vi "FormMain.vi"() -> ()   [LabVIEW 2018]
panel:
  out "String (transparent)":string
  in  "Vertical Add Button":bool
  in  "Vertical Open Button":bool
  in  "Vertical Stop Button":bool
  in  "Vertical Start Button":bool
  out "滑动杆":u8(slide) max=1 scale=0.0..15.0
  in  "TDMS Files Path":path
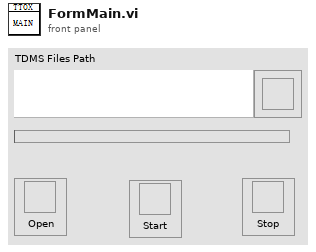
[diagram p1: front panel]
types:
  T1 = enum8{"Enabled", "Disabled", "Disabled and Grayed Out"}
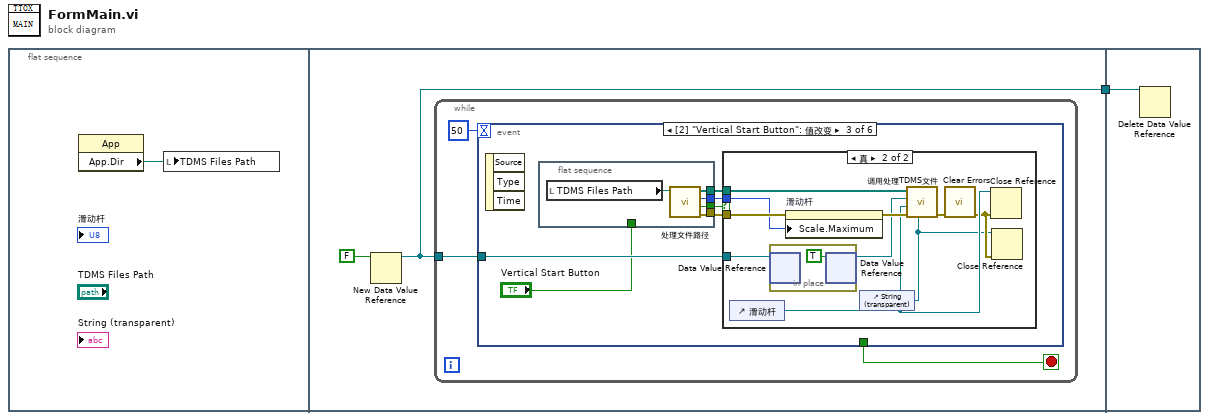
[diagram p0: block diagram]
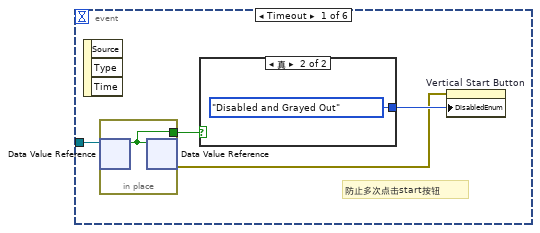
[diagram p2: hidden frame]
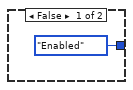
[diagram p3: hidden frame]
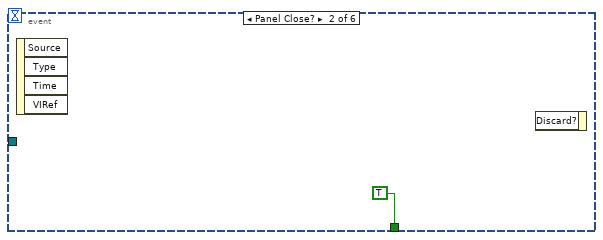
[diagram p4: hidden frame]
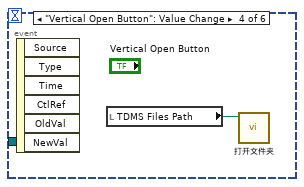
[diagram p6: hidden frame]
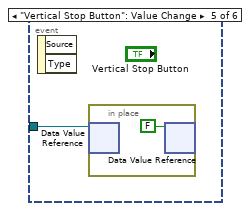
[diagram p7: hidden frame]
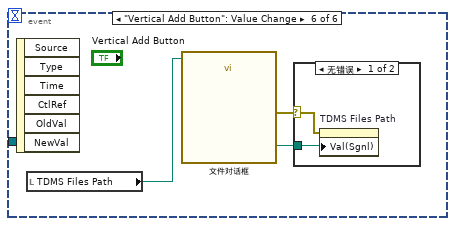
[diagram p8: hidden frame]
diagram:
  n1 = flat-sequence {
    tunnel: [w3] -> w1
    tunnel: w1 -> [w46]
    frame #0 {
      n2 = property class="App"() -> ("App.Dir"=w2:path)  [unwired: 2 in, 2 out]
      n3 = local write "TDMS Files Path"(w2) -> ()
    }
    frame #1 {
      n4 = New Data Value Reference(data value=FALSE) -> (data value reference=w3:refnum<data-value>)  [unwired: 1 in, 1 out]
      n5 = while {
        tunnel: w3 -> [w7]
        stop <- w6 stop-if-true
        n6 = event shown="[2] \"Vertical Start Button\": 值改变" {
          selector: _ -> [_ _ _ _ _ _]
          dyn-events: _ -> [_ _ _ _ _ _]
          timeout: 50 -> [_ _ _ _ _ _]
          tunnel: w7 -> [w11 _ w18 _ w39 _]
          tunnel: [_ TRUE _ _ _ _] -> w6
          event Timeout {
            # "防止多次点击start按钮"
            n7 = event-data() -> ()  [unwired: 1 in, 3 out]
            n8 = in-place {
              in-place-border: [w14] -> w10
              n9 = in-place-dvr #1(w11) -> (w14:bool)  [unwired: 1 out]
              n10 = in-place-dvr #1(w14) -> (w8:errorcluster)  [unwired: 1 out]
            }
            n11 = case shown="真" w10 {
              tunnel: [T1."Enabled" ("禁用") T1."Disabled and Grayed Out" ("禁用")] -> w9
              frame False {
              }
              frame True {
              }
            }
            n12 = property on="Vertical Start Button" class="Bool"(error in=w8, "DisabledEnum"=w9) -> ()  [unwired: 1 in, 2 out]
          }
          event Panel Close? {
            n13 = event-data() -> ()  [unwired: 1 in, 4 out]
            n14 = event-data() -> ()  [unwired: 2 in, 1 out]
          }
          event "Vertical Start Button": Value Change {
            n15 = event-data() -> ()  [unwired: 1 in, 3 out]
            n16 = flat-sequence {
              tunnel: [w25] -> w21
              tunnel: [w24] -> w20
              tunnel: [w23] -> w19
              tunnel: "Vertical Start Button" -> [_]
              tunnel: [w22] -> w16
              frame #0 {
                n17 = local read "TDMS Files Path"() -> (w26:path)
                n18 = call "处理文件路径.vi"("TDMS Files Path"=w26) -> ("错误输出"=w24:errorcluster, "可用"=w25:bool, "文件个数"=w22:i32, "文件数组"=w23:path[])  [unwired: 7 in]
              }
            }
            n19 = case shown="真" w21 {
              tunnel: w20 -> [_ w36]
              tunnel: w19 -> [_ w35]
              tunnel: w18 -> [_ w33]
              tunnel: w16 -> [_ w30]
              frame False {
              }
              frame True {
                n20 = control-ref of="滑动杆"() -> (w29:refnum<vi>)
                n21 = in-place {
                  n22 = in-place-dvr #2(w33) -> ()  [unwired: 2 out]
                  n23 = in-place-dvr #2(TRUE ("数据值")) -> (w32:refnum<data-value>)  [unwired: 1 out]
                }
                n24 = property on="滑动杆" class="Slide (严格)"(error in=w36, "Scale.Maximum"=w30) -> (error out=w34:errorcluster)  [unwired: 1 in, 1 out]
                n25 = control-ref of="String (transparent)"() -> (w27:refnum<vi>)
                n26 = call "调用处理TDMS文件.vi"("String"=w27, "error in (no error)"=w34, "滑动杆引用"=w29, "停止引用"=w32, "文件路径数组"=w35) -> ("error out"=w31:errorcluster)  [unwired: 6 in]
                n27 = call <vilib>:"Clear Errors.vi"("error in (no error)"=w31) -> ("error out"=w28:errorcluster)  [unwired: 5 in, 1 out]
                n28 = Close Reference(reference=w29, error in (no error)=w28) -> ()  [unwired: 1 out]
                n29 = Close Reference(reference=w27, error in (no error)=w28) -> ()  [unwired: 1 out]
              }
            }
          }
          event "Vertical Open Button": Value Change {
            n30 = event-data() -> ()  [unwired: 1 in, 6 out]
            n31 = local read "TDMS Files Path"() -> (w38:path)
            n32 = call "打开文件夹.vi"("文件夹"=w38) -> ()  [unwired: 10 in, 1 out]
          }
          event "Vertical Stop Button": Value Change {
            n33 = event-data() -> ()  [unwired: 1 in, 2 out]
            n34 = in-place {
              n35 = in-place-dvr #3(w39) -> ()  [unwired: 2 out]
              n36 = in-place-dvr #3(FALSE ("数据值")) -> ()  [unwired: 2 out]
            }
          }
          event "Vertical Add Button": Value Change {
            n37 = event-data() -> ()  [unwired: 1 in, 6 out]
            n38 = local read "TDMS Files Path"() -> (w42:path)
            n39 = call "文件对话框"("start path"=w42) -> ("selected path"=w43:path, "error out"=w41:errorcluster)  [unwired: 11 in, 2 out]
            n40 = case shown="无错误" w41 {
              selector: w41 -> [w44 _]
              tunnel: w43 -> [w45 _]
              frame No Error {
                n41 = property on="TDMS Files Path" class="Path"(error in=w44, "Val(Sgnl)"=w45) -> ()  [unwired: 1 in, 2 out]
              }
              frame Error {
              }
            }
          }
        }
      }
    }
    frame #2 {
      n42 = Delete Data Value Reference(data value reference=w46) -> ()  [unwired: 1 in, 2 out]
    }
  }
